vi "Periodic Tasks.vi"(8 "error in":errorcluster) -> ()   [LabVIEW 2014]
doc: "This VI runs in parallel to other tasks. It can contain as many user-defined periodic loops as you need. These can carry out PID or other sorts of timed response."
uses:
  <vilib>/Rock Robotics/WPI/Relay/WPI_RelayValue.ctl
  <vilib>/Rock Robotics/WPI/Solenoid/WPI_SolenoidValue.ctl
  Support Files/Global Data!!!.vi
  <vilib>/Rock Robotics/WPI/Solenoid/WPI_SolenoidSetEnum.vi
  <vilib>/Rock Robotics/Network Tables/SD Write Number.vi
panel:
  # "Only need one"
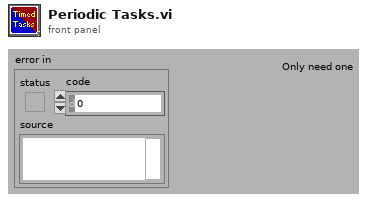
[diagram p1: front panel]
types:
  T1 = typedef "WPI_RelayValue.ctl" = enum16{"Off", "On", "Forward", "Reverse"}
  T2 = typedef "WPI_SolenoidDevRef.ctl" = cluster{"DevStatus":errorcluster, "Pneumatics Control Module":u8, "Forward Solenoid Channel":T3, "Reverse Solenoid Channel":T3}
  T3 = typedef "WPI_SolenoidChannel.ctl" = enum8{"Solenoid 0", "Solenoid 1", "Solenoid 2", "Solenoid 3", "Solenoid 4", "Solenoid 5", "Solenoid 6", "Solenoid 7", "Invalid"}
  T4 = typedef "WPI_DigitalInputDevRef.ctl" = cluster{"DevStatus":errorcluster, "DIO Channel":T5, "Controller":T6}
  T5 = typedef "FPGA_DIOChannel.ctl" = enum8{"DIO 0", "DIO 1", "DIO 2", "DIO 3", "DIO 4", "DIO 5", "DIO 6", "DIO 7", "DIO 8", "DIO 9", "DIO MXP 0", "DIO MXP 1", "DIO MXP 2", "DIO MXP 3", "DIO MXP 4", "DIO MXP 5", "DIO MXP 6", "DIO MXP 7", "DIO MXP 8", "DIO MXP 9", "DIO MXP 10", "DIO MXP 11", "DIO MXP 12", "DIO MXP 13", "DIO MXP 14", "DIO MXP 15", "Invalid"}
  T6 = typedef "FPGA_TypedefDigitalModule.ctl" = enum16{"Controller 1"}
  T7 = typedef "WPI_SolenoidValue.ctl" = enum16{"Off", "On", "Forward", "Reverse"}
  T8 = typedef "WPI_MotorControlDeviceRef.ctl" = cluster{"DeviceStatus":errorcluster, "Type":T9, "PWM":cluster{"Controller":T6, "PWM Channel":T10, "DeadBand":T11}, "CAN":cluster{"Device Number":u8, "Control Mode":T12, "Semaphore":T13, "Max Vout":dbl, "TalonSRX Control Mode":T14}, "Invert":bool, "TransformRef":T15, "InvTransformRef":T15}
  T9 = typedef "WPI_MotorControlType.ctl" = enum16{"PWM", "CAN", "CANTalonSRX"}
  T10 = typedef "FPGA_DIOPWMChannel.ctl" = enum8{"PWM 0", "PWM 1", "PWM 2", "PWM 3", "PWM 4", "PWM 5", "PWM 6", "PWM 7", "PWM 8", "PWM 9", "PWM MXP 0", "PWM MXP 1", "PWM MXP 2", "PWM MXP 3", "PWM MXP 4", "PWM MXP 5", "PWM MXP 6", "PWM MXP 7", "PWM MXP 8", "PWM MXP 9", "Invalid"}
  T11 = typedef "WPI_PWMDeadband.ctl" = cluster{"Name":string, "maxPositivePwm":i32, "minPositivePwm":i32, "centerPwm":i32, "maxNegativePwm":i32, "minNegativePwm":i32, "angularRange":u16}
  T12 = typedef "WPI_CANJaguar_ControlMode.ctl" = enum8{"Percent VBus", "Current", "Speed", "Position", "Voltage"}
  T13 = typedef "Semaphore RefNum" = refnum<k1>
  T14 = typedef "WPI_CANTalonSRX_APIControlMode.ctl" = enum8{"Percent VBus", "Speed", "Position", "Slave", "Unchanged / Invalid"}
  T15 = typedef "WPI_PWMTransform_ConPane.ctl" = refnum<vi>
  T16 = typedef "WPI_GyroDevRef.ctl" = cluster{"DevStatus":errorcluster, "Analog Module":T17, "Analog Channel":T18, "Offset":dbl, "Gain (VoltsPerDegree/Second)":dbl}
  T17 = typedef "FPGA_TypedefAnalogModule.ctl" = enum16{"Controller 1"}
  T18 = typedef "FPGA_AIChannel.ctl" = enum8{"AI 0", "AI 1", "AI 2", "AI 3", "AI MXP 0", "AI MXP 1", "AI MXP 2", "AI MXP 3", "Invalid"}
  T19 = typedef "WPI_EncoderDevRef.ctl" = cluster{"DevStatus":errorcluster, "EncoderIndex":T20, "CounterIndex":T21, "DistancePerCount":dbl, "Decoding Type":T22}
  T20 = typedef "FPGA_EncoderIdx.ctl" = enum8{"Enc 0", "Enc 1", "Enc 2", "Enc 3", "Enc 4", "Enc 5", "Enc 6", "Enc 7", "Invalid"}
  T21 = typedef "FPGA_CounterCtrSystemIndex.ctl" = enum8{"Ctr 0", "Ctr 1", "Ctr 2", "Ctr 3", "Ctr 4", "Ctr 5", "Ctr 6", "Ctr 7", "Invalid"}
  T22 = typedef "WPI_EncoderType.ctl" = enum16{"1x", "2x", "4x"}
  T23 = typedef "WPI_RelayDevRef.ctl" = cluster{"DevStatus":errorcluster, "Relay Channel":T24, "Controller":T6, "Relay Direction":T25}
  T24 = typedef "FPGA_DIORelayChannel.ctl" = enum8{"Relay 0", "Relay 1", "Relay 2", "Relay 3", "Invalid"}
  T25 = typedef "WPI_RelayDirection.ctl" = enum16{"Both directions", "Forward only", "Reverse only"}
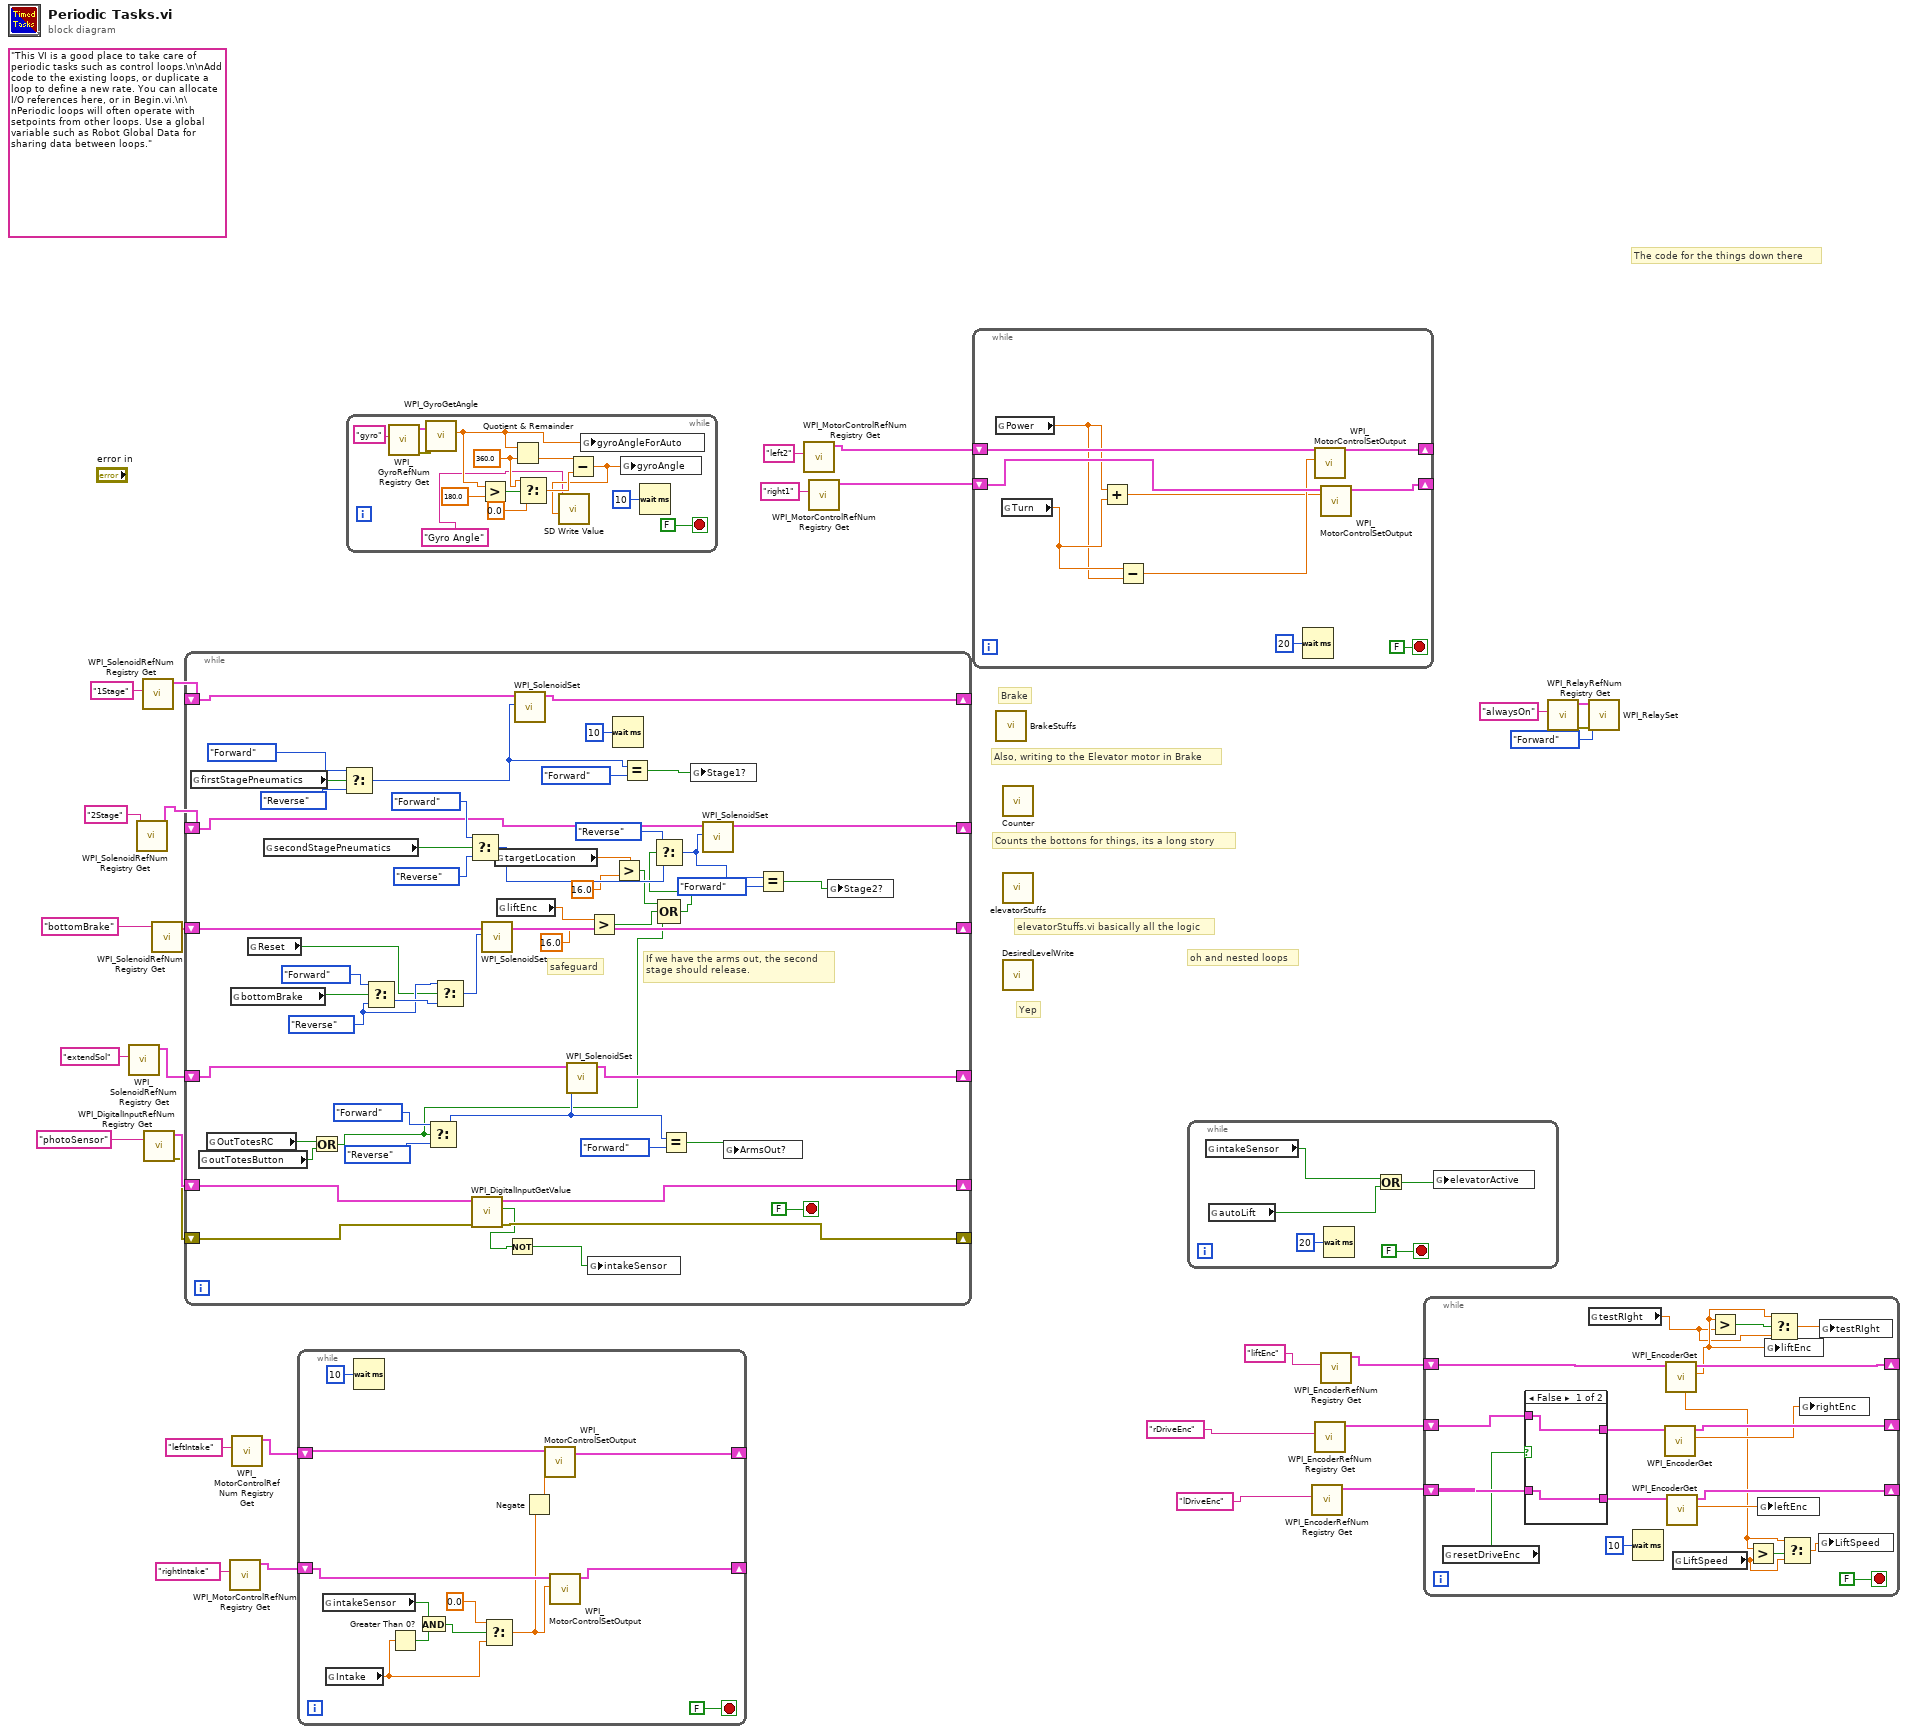
[diagram p0: block diagram]
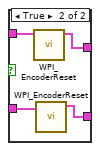
[diagram p2: hidden frame]
diagram:
  (unwired) "This VI is a good place to take care of periodic tasks such as control loops.\n\nAdd code to the existing loops, or duplicate a loop to define a new rate. You can allocate I/O references here, or in Begin.vi.\n\nPeriodic loops will often operate with setpoints from other loops. Use a global variable such as Robot Global Data for sharing data between loops."
  # "Yep"
  # "Counts the bottons for things, its a long story"
  # "oh and nested loops"
  # "elevatorStuffs.vi basically all the logic"
  # "Also, writing to the Elevator motor in Brake"
  # "Brake"
  # "The code for the things down there"
  n1 = call <vilib>:"WPI_SolenoidRefNum Registry Get.vi"("refnum name"="extendSol") -> ("SolenoidDevRef"=w10:T2)  [unwired: 9 in, 1 out]
  n2 = call <vilib>:"WPI_SolenoidRefNum Registry Get.vi"("refnum name"="2Stage") -> ("SolenoidDevRef"=w22:T2)  [unwired: 9 in, 1 out]
  n3 = call <vilib>:"WPI_SolenoidRefNum Registry Get.vi"("refnum name"="1Stage") -> ("SolenoidDevRef"=w21:T2)  [unwired: 9 in, 1 out]
  n4 = call <vilib>:"WPI_DigitalInputRefNum Registry Get.vi"("refnum name"="photoSensor") -> ("error out"=w12:errorcluster, "DigitalInputDevRef"=w13:T4)  [unwired: 9 in]
  n5 = call <vilib>:"WPI_SolenoidRefNum Registry Get.vi"("refnum name"="bottomBrake") -> ("SolenoidDevRef"=w25:T2)  [unwired: 9 in, 1 out]
  n6 = while {
    shift-right: [w68] -> _
    shift-left: w25 -> [w67]
    shift-right: [w69] -> _
    shift-left: w21 -> [w70]
    shift-right: [w53] -> _
    shift-left: w22 -> [w52]
    shift-right: [w64] -> _
    shift-left: w13 -> [w66]
    shift-right: [w63] -> _
    shift-left: w12 -> [w65]
    shift-right: [w60] -> _
    shift-left: w10 -> [w61]
    stop <- FALSE stop-if-true
    w72 = WPI_SolenoidValue."Reverse" ("f")
    # "If we have the arms out, the second\nstage should release."
    # "safeguard"
    n7 = global read "Global Data!!!.vi" "firstStagePneumatics"() -> (w55:bool)
    n8 = global read "Global Data!!!.vi" "outTotesButton"() -> (w32:bool)
    n9 = global read "Global Data!!!.vi" "OutTotesRC"() -> (w31:bool)
    n10 = global read "Global Data!!!.vi" "bottomBrake"() -> (w76:bool)
    n11 = global read "Global Data!!!.vi" "Reset"() -> (w71:bool)
    n12 = global read "Global Data!!!.vi" "secondStagePneumatics"() -> (w54:bool)
    n13 = Or(x=w31, y=w32) -> (x .or. y?=w30:bool)
    n14 = Select(t=WPI_SolenoidValue."Forward" ("Value"), s=w55, f=WPI_SolenoidValue."Reverse") -> (s? t:f=w39:T7)
    n15 = Select(t=WPI_SolenoidValue."Forward" ("f"), s=w76, f=w72) -> (s? t:f=w74:T7)
    n16 = Select(t=WPI_SolenoidValue."Forward" ("Value"), s=w30, f=WPI_SolenoidValue."Reverse") -> (s? t:f=w34:T7)
    n17 = Select(t=w72, s=w71, f=w74) -> (s? t:f=w73:T7)
    n18 = Select(t=WPI_SolenoidValue."Forward" ("Value"), s=w54, f=WPI_SolenoidValue."Reverse") -> (s? t:f=w51:T7)
    n19 = call <vilib>:"WPI_DigitalInputGetValue.vi"("error in (no error)"=w65, "DigitalInputDevRef"=w66) -> ("error out"=w63:errorcluster, "Value"=w62:bool, "DigitalInputDevRef"=w64:T4)  [unwired: 7 in]
    n20 = call-poly <vilib>:"WPI_SolenoidSet.vi"("Value"=w73, "SolenoidDevRef"=w67) -> ("SolenoidDevRef"=w68:T2)  [unwired: 8 in, 1 out]
    n21 = global read "Global Data!!!.vi" "targetLocation"() -> (w50:dbl)
    n22 = global read "Global Data!!!.vi" "liftEnc"() -> (w47:dbl)
    n23 = Not(x=w62) -> (.not. x?=w33:bool)
    n24 = call-poly <vilib>:"WPI_SolenoidSet.vi"("Value"=w39, "SolenoidDevRef"=w70) -> ("SolenoidDevRef"=w69:T2)  [unwired: 8 in, 1 out]
    n25 = call-poly <vilib>:"WPI_SolenoidSet.vi"("Value"=w34, "SolenoidDevRef"=w61) -> ("SolenoidDevRef"=w60:T2)  [unwired: 8 in, 1 out]
    n26 = global write "Global Data!!!.vi" "intakeSensor"(w33) -> ()
    n27 = Greater?(x=w47, y=16.0) -> (0:w43:bool)
    n28 = Wait (ms)(milliseconds to wait=u32 10) -> ()  [unwired: 1 out]
    n29 = Greater?(x=w50, y=16.0) -> (0:w44:bool)
    n30 = Equal?(x=w39, y=WPI_SolenoidValue."Forward") -> (x = y?=w37:bool)
    n31 = Compound Arithmetic op=OR(w44, w43, w30) -> (w45:bool)
    n32 = Select(t=WPI_SolenoidValue."Reverse", s=w45, f=w51) -> (s? t:f=w42:T7)
    n33 = Equal?(x=w34, y=WPI_SolenoidValue."Forward") -> (x = y?=w36:bool)
    n34 = global write "Global Data!!!.vi" "Stage1?"(w37) -> ()
    n35 = call-poly <vilib>:"WPI_SolenoidSet.vi"("Value"=w42, "SolenoidDevRef"=w52) -> ("SolenoidDevRef"=w53:T2)  [unwired: 8 in, 1 out]
    n36 = global write "Global Data!!!.vi" "ArmsOut?"(w36) -> ()
    n37 = Equal?(x=w42, y=WPI_SolenoidValue."Forward") -> (x = y?=w38:bool)
    n38 = global write "Global Data!!!.vi" "Stage2?"(w38) -> ()
  }
  n39 = call <vilib>:"WPI_MotorControlRefNum Registry Get.vi"("refnum name"="rightIntake") -> ("MotorControlDevRef"=w3:T8)  [unwired: 9 in, 1 out]
  n40 = call <vilib>:"WPI_MotorControlRefNum Registry Get.vi"("refnum name"="leftIntake") -> ("MotorControlDevRef"=w4:T8)  [unwired: 9 in, 1 out]
  n41 = while {
    shift-right: [w89] -> _
    shift-left: w4 -> [w92]
    shift-right: [w90] -> _
    shift-left: w3 -> [w91]
    stop <- FALSE stop-if-true
    n42 = global read "Global Data!!!.vi" "intakeSensor"() -> (w84:bool)
    n43 = global read "Global Data!!!.vi" "Intake"() -> (w82:dbl)
    n44 = Wait (ms)(milliseconds to wait=u32 10) -> ()  [unwired: 1 out]
    n45 = Greater Than 0?(x=w82) -> (x > 0?=w83:bool)
    n46 = And(x=w84, y=w83) -> (x .and. y?=w81:bool)
    n47 = Select(t=0.0, s=w81, f=w82) -> (s? t:f=w86:dbl)
    n48 = Negate(x=w86) -> (-x=w85:dbl)
    n49 = call <vilib>:"WPI_MotorControlSetOutput.vi"("Output"=w85, "MotorControlDevRef"=w92) -> ("MotorControlDevRef"=w89:T8)  [unwired: 7 in, 2 out]
    n50 = call <vilib>:"WPI_MotorControlSetOutput.vi"("Output"=w86, "MotorControlDevRef"=w91) -> ("MotorControlDevRef"=w90:T8)  [unwired: 7 in, 2 out]
  }
  n51 = while {
    stop <- FALSE stop-if-true
    w101 = 360.0 ("y")
    n52 = call <vilib>:"WPI_GyroRefNum Registry Get.vi"("refnum name"="gyro") -> ("error out"=w107:errorcluster, "GyroDevRef"=w106:T16)  [unwired: 9 in]
    n53 = call <vilib>:"WPI_GyroGetAngle.vi"("error in (no error)"=w107, "GyroDevRef"=w106) -> ("Angle"=w96:dbl)  [unwired: 6 in, 3 out]
    n54 = Greater?(x=w96, y=180.0) -> (0:w103:bool)
    n55 = Quotient & Remainder(x=w96, y=w101) -> (floor(x/y)=w105:dbl)  [unwired: 1 out]
    n56 = Select(t=w101, s=w103, f=0.0) -> (s? t:f=w104:dbl)
    n57 = Subtract(x=w105, y=w104) -> (x-y=w95:dbl)
    n58 = call-poly <vilib>:"SD Write Value.vi"("Numeric"=w95, "Name"="Gyro Angle") -> ()  [unwired: 8 in, 2 out]
    n59 = global write "Global Data!!!.vi" "gyroAngleForAuto"(w96) -> ()
    n60 = global write "Global Data!!!.vi" "gyroAngle"(w95) -> ()
    n61 = Wait (ms)(milliseconds to wait=u32 10) -> ()  [unwired: 1 out]
  }
  n62 = call <vilib>:"WPI_MotorControlRefNum Registry Get.vi"("refnum name"="left2") -> ("MotorControlDevRef"=w18:T8)  [unwired: 9 in, 1 out]
  n63 = call <vilib>:"WPI_MotorControlRefNum Registry Get.vi"("refnum name"="right1") -> ("MotorControlDevRef"=w17:T8)  [unwired: 9 in, 1 out]
  n64 = while {
    shift-right: [w112] -> _
    shift-left: w18 -> [w113]
    shift-right: [w115] -> _
    shift-left: w17 -> [w114]
    stop <- FALSE stop-if-true
    n65 = global read "Global Data!!!.vi" "Power"() -> (w110:dbl)
    n66 = global read "Global Data!!!.vi" "Turn"() -> (w111:dbl)
    n67 = Add(x=w110, y=w111) -> (x+y=w108:dbl)
    n68 = Subtract(x=w111, y=w110) -> (x-y=w109:dbl)
    n69 = Wait (ms)(milliseconds to wait=u32 20) -> ()  [unwired: 1 out]
    n70 = call <vilib>:"WPI_MotorControlSetOutput.vi"("Output"=w109, "MotorControlDevRef"=w113) -> ("MotorControlDevRef"=w112:T8)  [unwired: 7 in, 2 out]
    n71 = call <vilib>:"WPI_MotorControlSetOutput.vi"("Output"=w108, "MotorControlDevRef"=w114) -> ("MotorControlDevRef"=w115:T8)  [unwired: 7 in, 2 out]
  }
  n72 = call "BrakeStuffs.vi"() -> ()  [unwired: 12 in]
  n73 = call "Counter.vi"() -> ()  [unwired: 12 in]
  n74 = call "elevatorStuffs.vi"() -> ()  [unwired: 11 in]
  n75 = call "DesiredLevelWrite.vi"() -> ()  [unwired: 12 in]
  n76 = while {
    stop <- FALSE stop-if-true
    n77 = global read "Global Data!!!.vi" "intakeSensor"() -> (w118:bool)
    n78 = global read "Global Data!!!.vi" "autoLift"() -> (w122:bool)
    n79 = Wait (ms)(milliseconds to wait=u32 20) -> ()  [unwired: 1 out]
    n80 = Or(x=w118, y=w122) -> (x .or. y?=w119:bool)
    n81 = global write "Global Data!!!.vi" "elevatorActive"(w119) -> ()
  }
  n82 = call <vilib>:"WPI_EncoderRefNum Registry Get.vi"("refnum name"="lDriveEnc") -> ("EncoderDevRef"=w27:T19)  [unwired: 9 in, 1 out]
  n83 = call <vilib>:"WPI_EncoderRefNum Registry Get.vi"("refnum name"="rDriveEnc") -> ("EncoderDevRef"=w28:T19)  [unwired: 9 in, 1 out]
  n84 = call <vilib>:"WPI_EncoderRefNum Registry Get.vi"("refnum name"="liftEnc") -> ("EncoderDevRef"=w29:T19)  [unwired: 9 in, 1 out]
  n85 = while {
    shift-right: [w143] -> _
    shift-left: w29 -> [w142]
    shift-right: [w141] -> _
    shift-left: w28 -> [w134]
    shift-right: [w140] -> _
    shift-left: w27 -> [w136]
    stop <- FALSE stop-if-true
    n86 = global read "Global Data!!!.vi" "resetDriveEnc"() -> (w132:bool)
    n87 = case shown="False" w132 {
      tunnel: w136 -> [w144 w149]
      tunnel: [w144 w148] -> w135
      tunnel: w134 -> [w145 w147]
      tunnel: [w145 w146] -> w133
      frame False {
      }
      frame True {
        n88 = call <vilib>:"WPI_EncoderReset.vi"("EncoderDevRef"=w147) -> ("EncoderDevRef"=w146:T19)  [unwired: 9 in, 1 out]
        n89 = call <vilib>:"WPI_EncoderReset.vi"("EncoderDevRef"=w149) -> ("EncoderDevRef"=w148:T19)  [unwired: 9 in, 1 out]
      }
    }
    n90 = global read "Global Data!!!.vi" "testRIght"() -> (w123:dbl)
    n91 = Wait (ms)(milliseconds to wait=u32 10) -> ()  [unwired: 1 out]
    n92 = call <vilib>:"WPI_EncoderGet.vi"("EncoderDevRef"=w133) -> ("Distance"=w131:dbl, "EncoderDevRef"=w141:T19)  [unwired: 5 in, 4 out]
    n93 = call <vilib>:"WPI_EncoderGet.vi"("EncoderDevRef"=w142) -> ("Distance"=w124:dbl, "EncoderDevRef"=w143:T19, "Rate"=w128:dbl)  [unwired: 5 in, 3 out]
    n94 = call <vilib>:"WPI_EncoderGet.vi"("EncoderDevRef"=w135) -> ("Distance"=w137:dbl, "EncoderDevRef"=w140:T19)  [unwired: 5 in, 4 out]
    n95 = global read "Global Data!!!.vi" "LiftSpeed"() -> (w127:dbl)
    n96 = Greater?(x=w124, y=w123) -> (0:w126:bool)
    n97 = Greater?(x=w128, y=w127) -> (0:w130:bool)
    n98 = global write "Global Data!!!.vi" "leftEnc"(w137) -> ()
    n99 = global write "Global Data!!!.vi" "liftEnc"(w124) -> ()
    n100 = Select(t=w124, s=w126, f=w123) -> (s? t:f=w125:dbl)
    n101 = Select(t=w128, s=w130, f=w127) -> (s? t:f=w129:dbl)
    n102 = global write "Global Data!!!.vi" "rightEnc"(w131) -> ()
    n103 = global write "Global Data!!!.vi" "LiftSpeed"(w129) -> ()
    n104 = global write "Global Data!!!.vi" "testRIght"(w125) -> ()
  }
  n105 = call <vilib>:"WPI_RelayRefNum Registry Get.vi"("refnum name"="alwaysOn") -> ("error out"=w8:errorcluster, "RelayDevRef"=w7:T23)  [unwired: 9 in]
  n106 = call <vilib>:"WPI_RelaySet.vi"("error in (no error)"=w8, "RelayValue"=WPI_RelayValue."Forward", "RelayDevRef"=w7) -> ()  [unwired: 7 in, 2 out]
